vi "sub_list cell color.vi"(8 "error in (no error)":errorcluster caption="错误输入（无错误）", 9 "Reset?(F)":bool, 10 "TR_Unit_Arr":T1[](array[typedef]), 11 "list ref":refnum<vi>) -> (0 "error out":errorcluster caption="错误输出", 3 "list ref out":refnum<vi>)   [LabVIEW 2011]
uses:
  _USB_CAN_T_R_Unit_.ctl
  <vilib>/Utility/miscctls.llb/LVRowAndColumnTypeDef.ctl
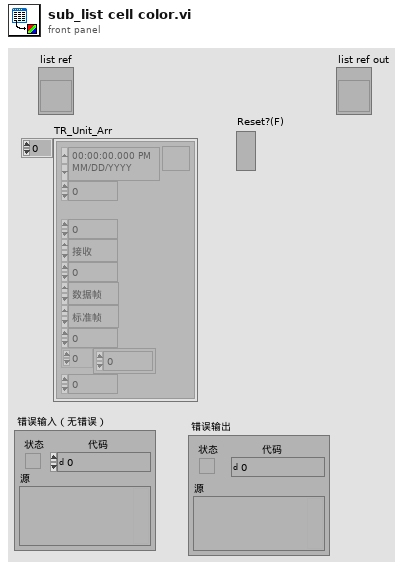
[diagram p1: front panel]
types:
  T1 = typedef "_USB_CAN_T_R_Unit_.ctl" = cluster{"time":timestamp, "channel":u16, "TimeStamp":u32, "tr":enum16{"接收", "发送"}, "id":u32, "Type":enum16{"数据帧", "远程帧"}, "Format":enum16{"标准帧", "扩展帧"}, "len":u8, "data":u8[], "sysTime":u32}
  T2 = typedef "LVRowAndColumnTypeDef.ctl" = cluster{"Row":i32, "Column":i32}
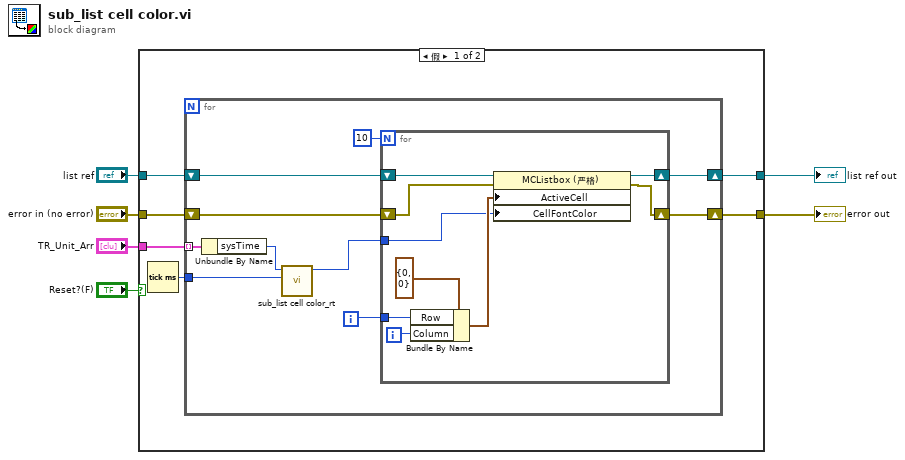
[diagram p0: block diagram]
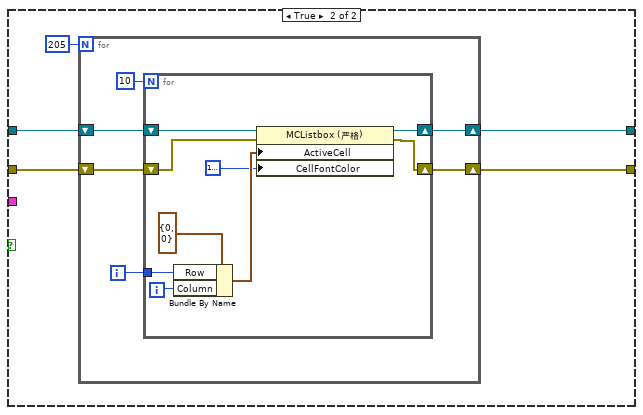
[diagram p2: hidden frame]
diagram:
  n1 = case shown="假" "Reset?(F)" {
    tunnel: "list ref" -> [w10 w35]
    tunnel: "error in (no error)" -> [w9 w34]
    tunnel: [w8 w33] -> w3
    tunnel: [w7 w32] -> w2
    tunnel: "TR_Unit_Arr" -> [w12 _]
    frame False {
      n2 = Tick Count (ms)() -> (millisecond timer value=w11:u32)
      n3 = for {
        tunnel: w12 -> [w22] mode=indexing
        tunnel: w11 -> [w20]
        shift-right: [w16] -> w8
        shift-left: w10 -> [w18]
        shift-right: [w15] -> w7
        shift-left: w9 -> [w17]
        i -> [w14]
        n4 = Unbundle By Name(w22) -> ("sysTime"=w21:u32)
        n5 = call "sub_list cell color_rt.vi"("millisecond timer"=w20, "sysTime"=w21) -> ("cell color"=w13:u32)  [unwired: 9 in]
        n6 = for {
          N: 10 -> [_]
          shift-right: [w30] -> w16
          shift-left: w18 -> [w31]
          shift-right: [w24] -> w15
          shift-left: w17 -> [w25]
          tunnel: w14 -> [w28]
          tunnel: w13 -> [w23]
          i -> [w27]
          n7 = Bundle By Name(cluster=T2 {"Row"=0, "Column"=0} ("活动单元格:活动单元格"), "Row"=w28, "Column"=w27) -> (w26:T2)
          n8 = property class="MCListbox (严格)"(reference=w31, error in=w25, "ActiveCell"=w26, "CellFontColor"=w23) -> (reference out=w30:refnum<vi>, error out=w24:errorcluster)
        }
      }
    }
    frame True {
      n9 = for {
        N: 205 -> [_]
        shift-right: [w39] -> w33
        shift-left: w35 -> [w41]
        shift-right: [w38] -> w32
        shift-left: w34 -> [w40]
        i -> [w37]
        n10 = for {
          N: 10 -> [_]
          shift-right: [w50] -> w39
          shift-left: w41 -> [w51]
          shift-right: [w44] -> w38
          shift-left: w40 -> [w45]
          tunnel: w37 -> [w48]
          i -> [w47]
          n11 = Bundle By Name(cluster=T2 {"Row"=0, "Column"=0} ("活动单元格:活动单元格"), "Row"=w48, "Column"=w47) -> (w46:T2)
          n12 = property class="MCListbox (严格)"(reference=w51, error in=w45, "ActiveCell"=w46, "CellFontColor"=u32 16777222) -> (reference out=w50:refnum<vi>, error out=w44:errorcluster)
        }
      }
    }
  }
  "error out" <- w2
  "list ref out" <- w3
